vi "Not A Refnum (Text).vi"(8 "error in (no error)":errorcluster, 11 "Text Log File in":refnum<class "Text Log File.lvclass">) -> (0 "error out":errorcluster, 2 "Not a Refnum?":bool, 3 "Text Log File out":refnum<class "Text Log File.lvclass">)   [LabVIEW 2015, in "Text Log File.lvclass"]
uses:
  Text Log File.lvclass
  Text Log File.lvclass/Text Log File.ctl
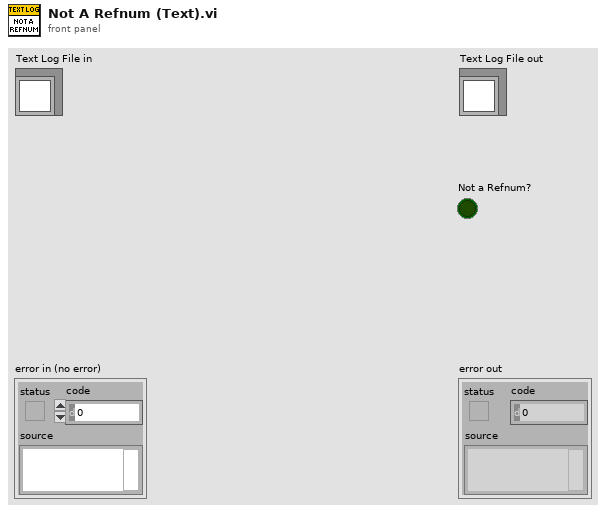
[diagram p1: front panel]
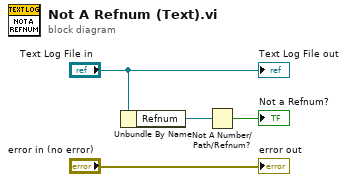
[diagram p0: block diagram]
diagram:
  n1 = Unbundle By Name("Text Log File in") -> ("Refnum"=w2:refnum<file>)
  n2 = Not A Number/Path/Refnum?(number/path/refnum=w2) -> (NaN/Path/Refnum?=→"Not a Refnum?":bool)
  "error out" <- "error in (no error)"
  "Text Log File out" <- "Text Log File in"
